vi "Global_external_move_cmd.vi"() -> ()   [LabVIEW 2018]
uses:
  Units_of_Move.ctl
panel:
  out "Goal Man Pos (Steps)":i32[](array[numeric])
  in  "Unit of Move":T1=1 items=["STEPS", "MICRONS / DEG", "MILLIMETER / DEG", "CENTIMETER / DEG", "INCHES / DEG"]
  in  "Rel Steps":string="10000"
  in  "Direction (+ true, - false)":bool
  in  "Motor":u16(ring)=2 items=["none", "1", "2", "3", "4", "all"]
  in  "external command":bool
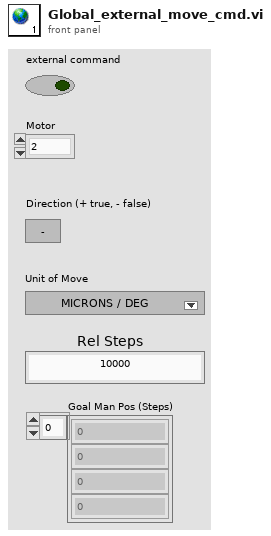
[diagram p1: front panel]
types:
  T1 = typedef "Units_of_Move.ctl" = u16
diagram:
